vi "Test Program.vi"() -> ()   [LabVIEW 2017]
uses:
  <vilib>/addons/RealSense/libRealSense3.lvlib
  <vilib>/vision/NI_Vision_Development_Module.lvlib
panel:
  out "Image":T1(plugin-control)
  out "error out":errorcluster
  out "Intensity Graph":sgl[][](graph)
  in  "stop":bool
  out "device count":i32
  # "All errors are #1, string is good"
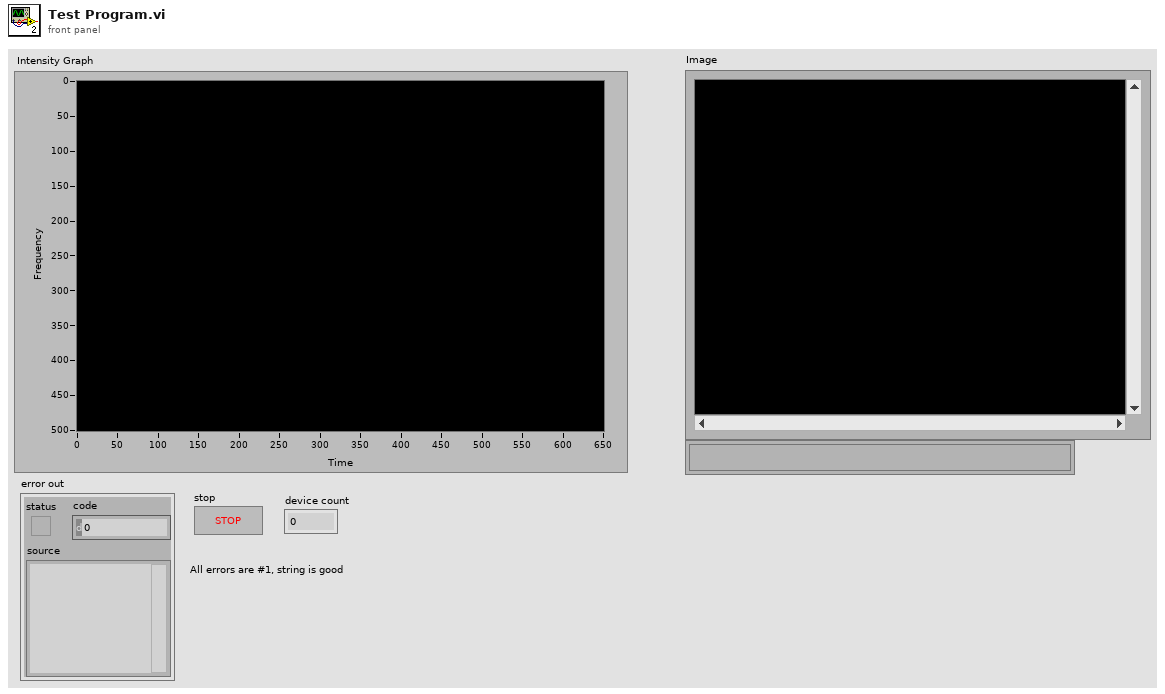
[diagram p1: front panel]
types:
  T1 = typedef "IMAQ Image.ctl" = refnum<image>
  T2 = typedef "Image Type" = u32
  T3 = cluster{"width":i32, "height":i32, "ppx":sgl, "ppy":sgl, "fx":sgl, "fy":sgl, "model":u32, "coeffs[0]":sgl, "coeffs[1]":sgl, "coeffs[2]":sgl, "coeffs[3]":sgl, "coeffs[4]":sgl}
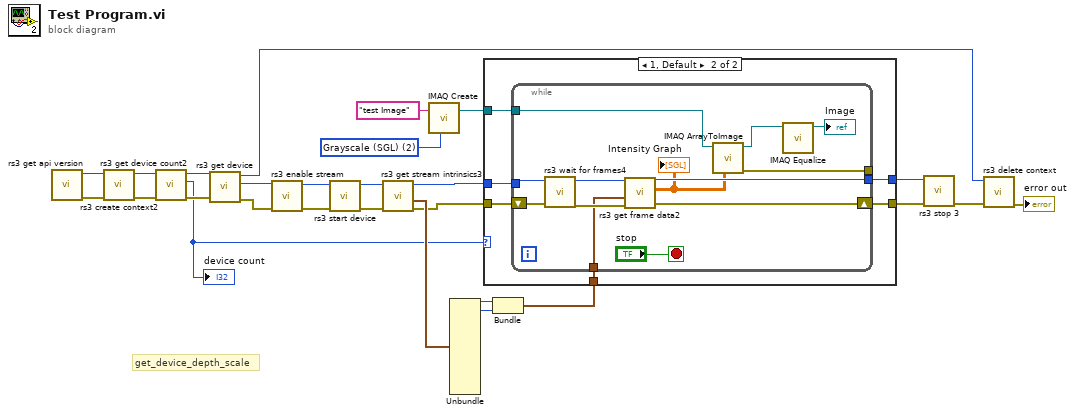
[diagram p0: block diagram]
diagram:
  w2 = T2 2 items=["Grayscale (U8)", "Grayscale (I16)", "Grayscale (SGL)", "Complex (CSG)", "RGB (U32)", "HSL (U32)", "RGB (U64)", "Grayscale (U16)"] ("Image Type")
  # "get_device_depth_scale"
  n1 = call <vilib>:"rs3 get api version.vi"() -> ("error out"=w16:errorcluster, "version"=w27:i32)  [unwired: 10 in]
  n2 = call <vilib>:"rs3 create context2.vi"("error in (no error)"=w16, "version"=w27) -> ("error out"=w15:errorcluster, "context"=w26:u32)  [unwired: 8 in]
  n3 = call <vilib>:"rs3 get device count2.vi"("error in"=w15, "context"=w26) -> ("error out"=w14:errorcluster, "count"=w5:i32, "context"=w25:u32)  [unwired: 7 in]
  "device count" <- w5
  n4 = call <vilib>:"rs3 get device.vi"("error in"=w14, "context"=w25) -> ("error out"=w13:errorcluster, "device"=w24:u32, "context"=w17:u64)  [unwired: 7 in]
  n5 = call <vilib>:"rs3 enable stream.vi"("error in"=w13, "device"=w24) -> ("error out"=w12:errorcluster, "device"=w23:u32)  [unwired: 8 in]
  n6 = call <vilib>:"rs3 start device.vi"("error in"=w12, "device"=w23) -> ("error out"=w11:errorcluster, "device"=w22:u64)  [unwired: 8 in]
  n7 = call <vilib>:"rs3 get stream intrinsics3.vi"("error in (no error)"=w11, "device in"=w22) -> ("error out"=w10:errorcluster, "intrin out"=w20:T3, "device out"=w21:u64)  [unwired: 7 in]
  n8 = call "IMAQ Create"("Image Name"="test Image", "Image Type"=w2) -> ("New Image"=w1:T1)  [unwired: 3 in, 1 out]
  n9 = Unbundle(w20) -> ("width"=w8:i32, "height"=w7:i32)  [unwired: 10 out]
  n10 = Bundle("width"=w8, "height"=w7) -> (w6:cluster{"width":i32, "height":i32})  [unwired: 1 in]
  n11 = case shown="1, Default" w5 {
    tunnel: w21 -> [w29 w35]
    tunnel: [w29 w34] -> w19
    tunnel: w10 -> [w28 w33]
    tunnel: [w28 w32] -> w9
    tunnel: w6 -> [_ w31]
    tunnel: w1 -> [_ w30]
    frame 0 {
    }
    frame 1, Default {
      n12 = while {
        tunnel: w35 -> [w46]
        tunnel: [w44] -> w34
        shift-right: [w42] -> w32
        shift-left: w33 -> [w43]
        tunnel: w31 -> [w41]
        tunnel: w30 -> [w39]
        tunnel: [w38] -> _
        stop <- "stop" stop-if-true
        n13 = call <vilib>:"rs3 wait for frames4.vi"("error in (no error)"=w43, "device in"=w46) -> ("error out"=w48:errorcluster, "device out"=w45:u64)  [unwired: 8 in]
        n14 = call <vilib>:"rs3 get frame data2.vi"("error in (no error)"=w48, "size"=w41, "device in"=w45) -> ("error out"=w42:errorcluster, "2D Array Output"=w40:sgl[][], "device out"=w44:u64)  [unwired: 6 in]
        "Intensity Graph" <- w40
        n15 = call "IMAQ ArrayToImage"("Image Pixels (Float)"=w40, "Image"=w39) -> ("error out"=w38:errorcluster, "Image Out"=w37:T1)  [unwired: 8 in]
        n16 = call "IMAQ Equalize"("Image Src"=w37) -> ("Image Dst Out"=→"Image":T1)  [unwired: 9 in, 1 out]
      }
    }
  }
  n17 = call <vilib>:"rs3 stop 3.vi"("error in (no error)"=w9, "device"=w19) -> ("error out"=w18:errorcluster)  [unwired: 8 in, 1 out]
  n18 = call <vilib>:"rs3 delete context.vi"("error in (no error)"=w18, "context"=w17) -> ("error out"=→"error out":errorcluster)  [unwired: 9 in]
